vi "Upload Firmware.vi"(5 "Progress Bar":refnum<vi>, 7 "COM Port":refnum<visa-resource-name>="COM5", 8 "Error In":errorcluster, 9 "Firmware Index":u16(ring) items=["LINX -  Serial / USB", "LINX -  Serial / USB [Debug] "], 10 "Device Index":u16=1, 11 "Family Index":T1=1 items=["Arduino", "Digilent", "PJRC"]) -> (0 "Error Out":errorcluster={"status"=TRUE, "code"=-1073807346, "source"="VISA Open in LVH-LINX.lvlib:Upload Firmware.vi"}, 1 "Log Path":path)   [LabVIEW 2014, in "LMH-LINX.lvlib"]
uses:
  LMH-LINX.lvlib
  Type Defs/Device Family.ctl
  Type Defs/All Firmware Data FGV States.ctl
  <vilib>/regexp/Match Regular Expression.xnode
  <vilib>/MakerHub/Toolbox/LMH-Toolbox.lvlib
  Device/Device.lvlib
panel:
  out "Success?":bool
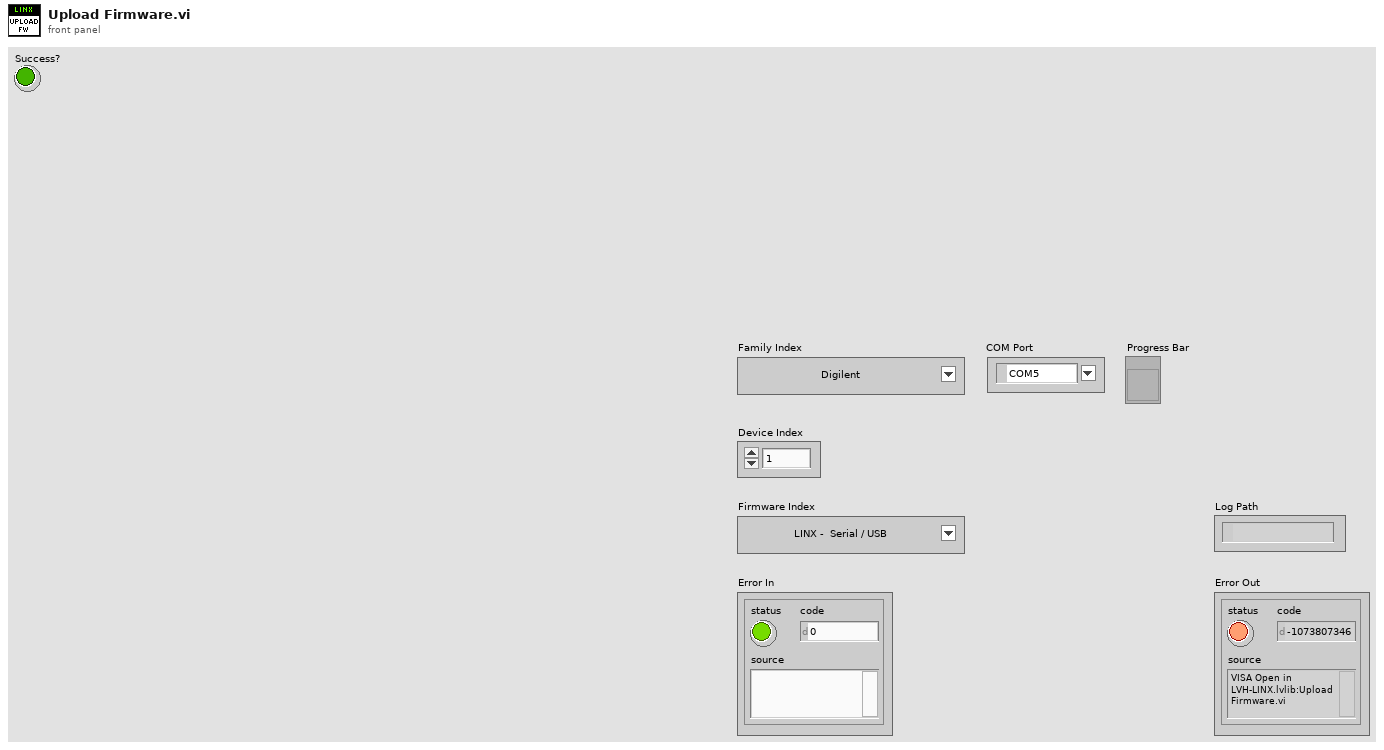
[diagram p1: front panel]
types:
  T1 = typedef "LMH-LINX.lvlib/Device Family.ctl" = u8
  T2 = typedef "LMH-LINX.lvlib/All Firmware Data FGV States.ctl" = enum16{"Set", "Get"}
  T3 = typedef "LMH-LINX.lvlib/Device Firmware.ctl" = cluster{"Firmware Name":string, "Firmware Path":path, "Description":string, "LINX Interface":string, "Flash Util Working Dir":path, "Flash Util Name":string, "Flash Util Args":string, "Flash Timeout (ms)":i32}
  T4 = typedef "LMH-LINX.lvlib/Device Data.ctl" = cluster{"Family ID":i32, "Family Name":string, "Device ID":i32, "Device Name":string, "Firmware Program Interfaces":string[], "Path":path}
  T5 = typedef "LVDateTimeRec.ctl" = cluster{"fractional second":dbl, "second":i32, "minute":i32, "hour":i32, "day of month":i32, "month":i32, "year":i32, "day of week":i32, "day of year":i32, "DST":i32}
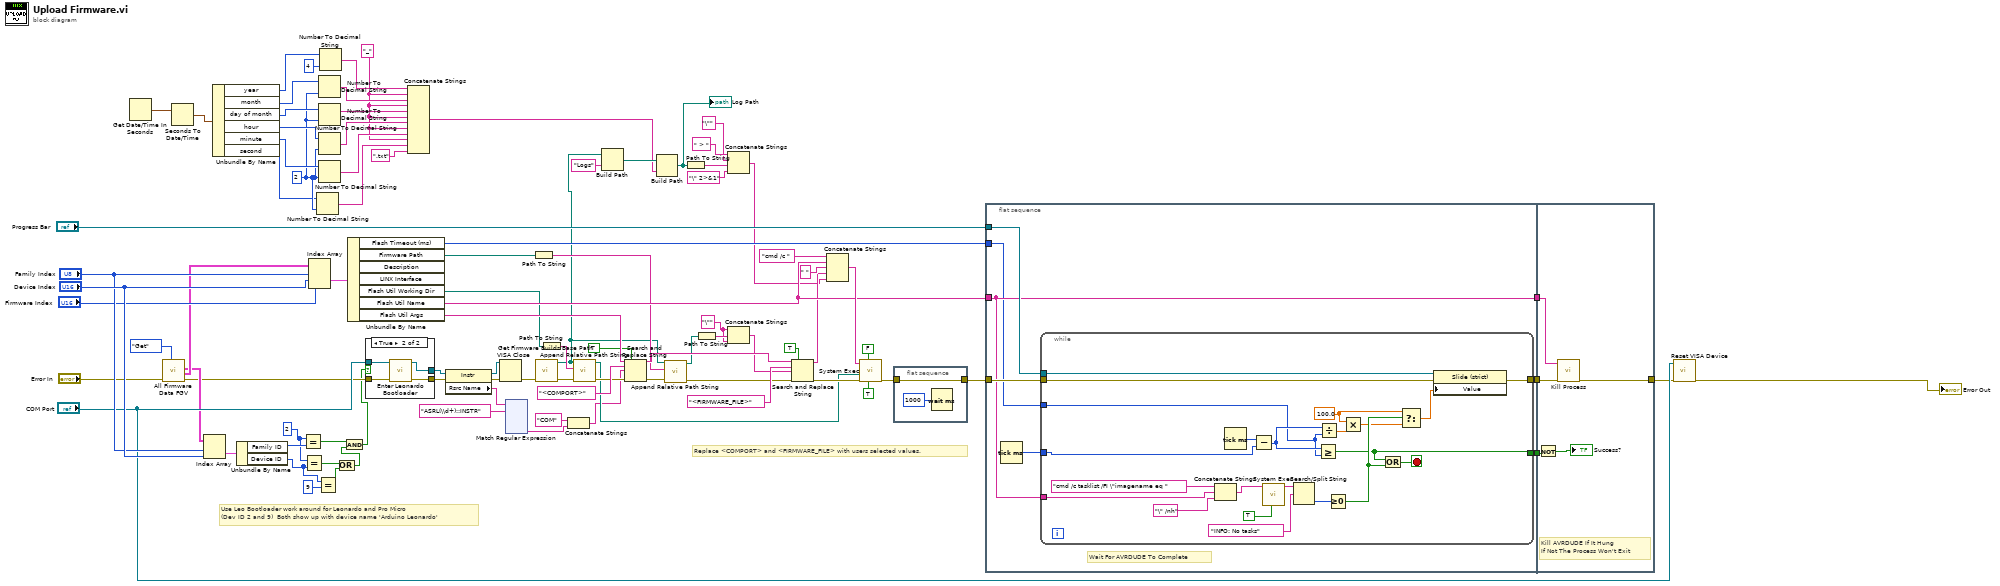
[diagram p0: block diagram]
diagram:
  w16 = "_" ("string")
  w20 = i16 2 ("width (-)")
  w47 = 2 ("x")
  w53 = "\"" ("string")
  # "Use Leo Bootloader work around for Leonardo and Pro Micro\n(Dev ID 2 and 9)  Both show up with device name 'Arduino Leonardo'"
  # "Replace <COMPORT> and <FIRMWARE_FILE> with users selected values."
  n1 = Get Date/Time In Seconds() -> (seconds since 1Jan1904=w36:timestamp)
  n2 = call "All Firmware Data FGV.vi"("All Firmware Data FGV States"=All_Firmware_Data_FGV_States."Get", "Error In"="Error In") -> ("Error Out"=w45:errorcluster, "Firmwares"=w83:T3[][][], "Devices"=w50:T4[][])  [unwired: 6 in, 1 out]
  n3 = Seconds To Date/Time(time stamp (now)=w36) -> (date time rec=w37:T5)  [unwired: 1 in]
  n4 = Index Array(array=w50, index (row)="Family Index", index (col)="Device Index") -> (element=w49:T4)
  n5 = Unbundle By Name(w37) -> ("year"=w35:i32, "month"=w34:i32, "day of month"=w33:i32, "hour"=w32:i32, "minute"=w31:i32, "second"=w19:i32)
  n6 = Unbundle By Name(w49) -> ("Family ID"=w48:i32, "Device ID"=w13:i32)
  n7 = Equal?(x=w47, y=w48) -> (x = y?=w46:bool)
  n8 = Equal?(x=w47, y=w13) -> (x = y?=w15:bool)
  n9 = Index Array(array=w83, index (dim 0)="Family Index", index (dim 1)="Device Index", index (dim 2)="Firmware Index") -> (element=w82:T3)
  n10 = Number To Decimal String(number=w19, width (-)=w20) -> (decimal integer string=w17:string)
  n11 = Equal?(x=w13, y=9 ("x")) -> (x = y?=w12:bool)
  n12 = Number To Decimal String(number=w34, width (-)=w20) -> (decimal integer string=w28:string)
  n13 = Number To Decimal String(number=w33, width (-)=w20) -> (decimal integer string=w27:string)
  n14 = Number To Decimal String(number=w32, width (-)=w20) -> (decimal integer string=w26:string)
  n15 = Number To Decimal String(number=w31, width (-)=w20) -> (decimal integer string=w25:string)
  n16 = Number To Decimal String(number=w35, width (-)=i16 4) -> (decimal integer string=w29:string)
  n17 = Or(x=w15, y=w12) -> (x .or. y?=w11:bool)
  n18 = And(x=w46, y=w11) -> (x .and. y?=w44:bool)
  n19 = Unbundle By Name(w82) -> ("Flash Timeout (ms)"=w51:i32, "Firmware Path"=w66:path, "Flash Util Working Dir"=w58:path, "Flash Util Name"=w70:string, "Flash Util Args"=w76:string)  [unwired: 2 out]
  n20 = case shown="True" w44 {
    tunnel: [w95 w100] -> w9
    tunnel: w45 -> [w95 w99]
    tunnel: [w96 w98] -> w10
    tunnel: "COM Port" -> [w96 w97]
    frame False {
    }
    frame True {
      n21 = call "Enter Leonardo Bootloader.vi"("Error In"=w99, "VISA resource name"=w97) -> ("Error Out"=w100:errorcluster, "VISA resource name"=w98:refnum<visa-resource-name>)  [unwired: 7 in, 1 out]
    }
  }
  n22 = Concatenate Strings(w29, w16, w28, w16, w27, w16, w26, w16, w25, w16, w17, ".txt" ("string")) -> (w24:string)
  n23 = property class="Instr"(reference=w10, error in=w9) -> (reference out=w7:refnum<visa-resource-name>, error out=w8:errorcluster, "Rsrc Name"=w4:string)
  n24 = VISA Close(VISA resource name=w7, error in (no error)=w8) -> (error out=w6:errorcluster)
  n25 = xnode "Match Regular Expression"("input string"=w4, "regular expression"="ASRL(\\d+)::INSTR") -> ("submatch 1"=w2:string)  [unwired: 4 in, 5 out]
  n26 = Path To String(path=w66) -> (string=w64:string)
  n27 = call "Get Firmware Builds Base Path.vi"("Error In"=w6) -> ("Error Out"=w60:errorcluster, "Firmware Builds Base Path"=w43:path)  [unwired: 9 in]
  n28 = Path To String(path=w58) -> (string=w57:string)
  n29 = Concatenate Strings("COM" ("string"), w2) -> (w1:string)
  n30 = call <vilib>:"Append Relative Path String.vi"("Error In"=w60, "Relative Path"=w57, "Base Path"=w43) -> ("Error Out"=w59:errorcluster, "Absolute Path"=w56:path)  [unwired: 7 in]
  n31 = Build Path(base path=w43, name or relative path="Logs") -> (appended path=w41:path)
  n32 = Search and Replace String(replace all?=TRUE ("replace all? (F)"), input string=w76, search string="<COMPORT>", replace string=w1, error in=w59) -> (result string=w67:string, error out=w52:errorcluster)  [unwired: 3 in, 2 out]
  n33 = Build Path(base path=w41, name or relative path=w24) -> (appended path=w40:path)
  "Log Path" <- w40
  n34 = call <vilib>:"Append Relative Path String.vi"("Error In"=w52, "Relative Path"=w64, "Base Path"=w43) -> ("Error Out"=w62:errorcluster, "Absolute Path"=w63:path)  [unwired: 7 in]
  n35 = Path To String(path=w40) -> (string=w23:string)
  n36 = Path To String(path=w63) -> (string=w54:string)
  n37 = Concatenate Strings(" > " ("string"), "\"" ("string"), w23, "\" 2>&1" ("string")) -> (w38:string)
  n38 = Concatenate Strings(w53, w54, w53) -> (w55:string)
  n39 = Search and Replace String(replace all?=TRUE ("replace all? (F)"), input string=w67, search string="<FIRMWARE_FILE>", replace string=w55, error in=w62) -> (result string=w65:string, error out=w61:errorcluster)  [unwired: 3 in, 2 out]
  n40 = Concatenate Strings("cmd /c " ("string"), w70, " " ("string"), w65, w38) -> (w73:string)
  n41 = call <vilib>:"System Exec.vi"("run minimized? (F)"=TRUE, "wait until completion? (T)"=FALSE, "error in (no error)"=w61, "working directory"=w56, "command line"=w73) -> ("error out"=w79:errorcluster)  [unwired: 3 in, 3 out]
  n42 = flat-sequence {
    tunnel: [w102] -> w71
    tunnel: w79 -> [w102]
    frame #0 {
      n43 = Wait (ms)(milliseconds to wait=u32 1000) -> ()  [unwired: 1 out]
    }
  }
  n44 = flat-sequence {
    tunnel: w71 -> [w107]
    tunnel: [w108] -> w87
    tunnel: "Progress Bar" -> [w106]
    tunnel: [w105] -> w86
    tunnel: w70 -> [w104]
    tunnel: [w104] -> w85
    tunnel: w51 -> [w103]
    tunnel: w87 -> [w136]
    tunnel: [w135] -> w72
    tunnel: w86 -> [w134]
    tunnel: w85 -> [w132]
    frame #0 {
      # "Wait For AVRDUDE To Complete"
      n45 = Tick Count (ms)() -> (millisecond timer value=w109:u32)
      n46 = while {
        tunnel: w109 -> [w130]
        tunnel: [w129] -> w108
        tunnel: w107 -> [w128]
        tunnel: w106 -> [w127]
        tunnel: [w115] -> w105
        tunnel: w104 -> [w111]
        tunnel: w103 -> [w110]
        stop <- w121 stop-if-true
        w118 = 100.0 ("x")
        n47 = Concatenate Strings("cmd /c tasklist /FI \"imagename eq " ("command line"), w111, "\" /nh" ("string")) -> (w113:string)
        n48 = Tick Count (ms)() -> (millisecond timer value=w131:u32)
        n49 = Subtract(x=w131, y=w130) -> (x-y=w126:u32)
        n50 = call <vilib>:"System Exec.vi"("run minimized? (F)"=TRUE, "command line"=w113) -> ("standard output"=w123:string)  [unwired: 6 in, 3 out]
        n51 = Search/Split String(string=w123, search string/char (-)="INFO: No tasks") -> (offset of match=w120:i32)  [unwired: 1 in, 2 out]
        n52 = Greater Or Equal?(x=w126, y=w110) -> (x >= y?=w115:bool)
        n53 = Divide(x=w126, y=w110) -> (x/y=w125:dbl)
        n54 = Greater Or Equal To 0?(x=w120) -> (x >= 0?=w119:bool)
        n55 = Multiply(x=w118, y=w125) -> (x*y=w117:dbl)
        n56 = Or(x=w115, y=w119) -> (x .or. y?=w121:bool)
        n57 = Select(t=w118, s=w119, f=w117) -> (s? t:f=w116:dbl)
        n58 = property class="Slide (strict)"(reference=w127, error in=w128, "Value"=w116) -> (error out=w129:errorcluster)  [unwired: 1 out]
      }
    }
    frame #1 {
      # "Kill AVRDUDE If It Hung\nIf Not The Process Won't Exit"
      n59 = Not(x=w134) -> (.not. x?=→"Success?":bool)
      n60 = call <vilib>:"Kill Process.vi"("Error In"=w136, "Process Name"=w132) -> ("Error Out"=w135:errorcluster)  [unwired: 9 in]
    }
  }
  n61 = call "Reset VISA Device.vi"("Error In"=w72, "VISA resource name"="COM Port") -> ("Error Out"=→"Error Out":errorcluster)  [unwired: 9 in]
